vi "InstrumentSetup.vi"() -> ()   [LabVIEW 2013, in "InstrControl.lvclass"]
uses:
  InstrControl.lvclass
  ArduinoControl/ArduinoControl.lvclass
  Switching/Switching.lvclass
panel:
  in  "WayneKerr 6425 Configurations":T1={"RC Configuration"=0, "AC amplitude [V]"=0.1, "AC frequency [Hz]"=1000, "GPIB Address"="23"} {"RC Configuration" items=["serial", "parallel"]}
  in  "MUX & Matrix Configurations":T2={"GPIB address"="10", "Matrix address"="1", "Mux1 address"="4", "Mux2 address"="5", "Matrix used?"=FALSE, "Switching"=refnum, "Matrix X Channels"={"Bias Supply / SMU LO"=5, "Bias Supply / SMU HI"=6, "CV Box LO"=3, "CV Box HI"=4, "CV Box LO IN"=7, "CV Box HI IN"=8, "Volt meter LO"=1, "Volt meter HI"=2, "Mux1 C1"=9, "Mux1 C2"=10, "Mux2 C1"=11, "Mux2 C2"=12}}
  in  "WayneKerr 6440B Configurations":T1={"RC Configuration"=0, "AC amplitude [V]"=0.1, "AC frequency [Hz]"=1000, "GPIB Address"="23"} {"RC Configuration" items=["serial", "parallel"]}
  in  "Keithley 2000 Configurations":T3={"Range"=0, "Range Value"=100.0, "Function"=3, "GPIB Address"="19"} {"Function" items=["AC Current", "DC Current", "AC Voltage", "DC Voltage", "2W-Resistance", "4W-Resistance", "Period", "Frequency", "Temperature", "Diode", "Continuity"]; "Range Value" format="%#.2g"; "Range" items=["Auto", "Manual"]}
  in  "Arduino Configuration":T4={"VISA address"="COM24", "T sensor"=enum."SHT", "Arduino"=refnum}
  in  "Keithley 487 Configurations":T5={"Compliance"=0, "Range:"=0, "GPIB Address"="22"} {"Range:" items=["Autorange", "2nA", "20nA", "200nA", "2 microAmp", "20 microAmp", "200 microAmp", "2 milliAmp"]; "Compliance" items=["20µA", "2mA"]}
  in  "Keithley 2410 Configurations":T6={"Current Limit"=0.0001, "GPIB Address"="24"}
  in  "Keithley 6517 Configurations":T7={"Current Limit"=1, "GPIB Address"="27"} {"Current Limit" items=["OFF", "ON"]}
  in  "Keithley 236/237 Configurations":T8={"current \ncompliance level"=0.0001, "compliance/\nmeasurement range (auto:0)"=6, "GPIB Address"="16"} {"compliance/\nmeasurement range (auto:0)" items=["auto / auto", "1 nA / 1.1 V", "10 nA / 11 V", "100 nA / 110 V", "0.001 mA / 110 V", "0.01 mA / 110 V", "0.1 mA / 110 V", "1 mA / 110 V", "10 mA / 110 V", "100 mA / 110 V"]; "current \ncompliance level" format="%.4f"}
  in  "Default GPIB addresses":T9={"KE 487"="22", "KE 6517"="27", "WK 6425"="17", "KE 236 SMU"="16", "HP 4263B"="18", "KE 2000"="19", "KE 2410"="24", "WK 6440B"="23", "Matrix"="10"}
  # "DEFAULT VALUES FOR INSTRUMENT SETUP"
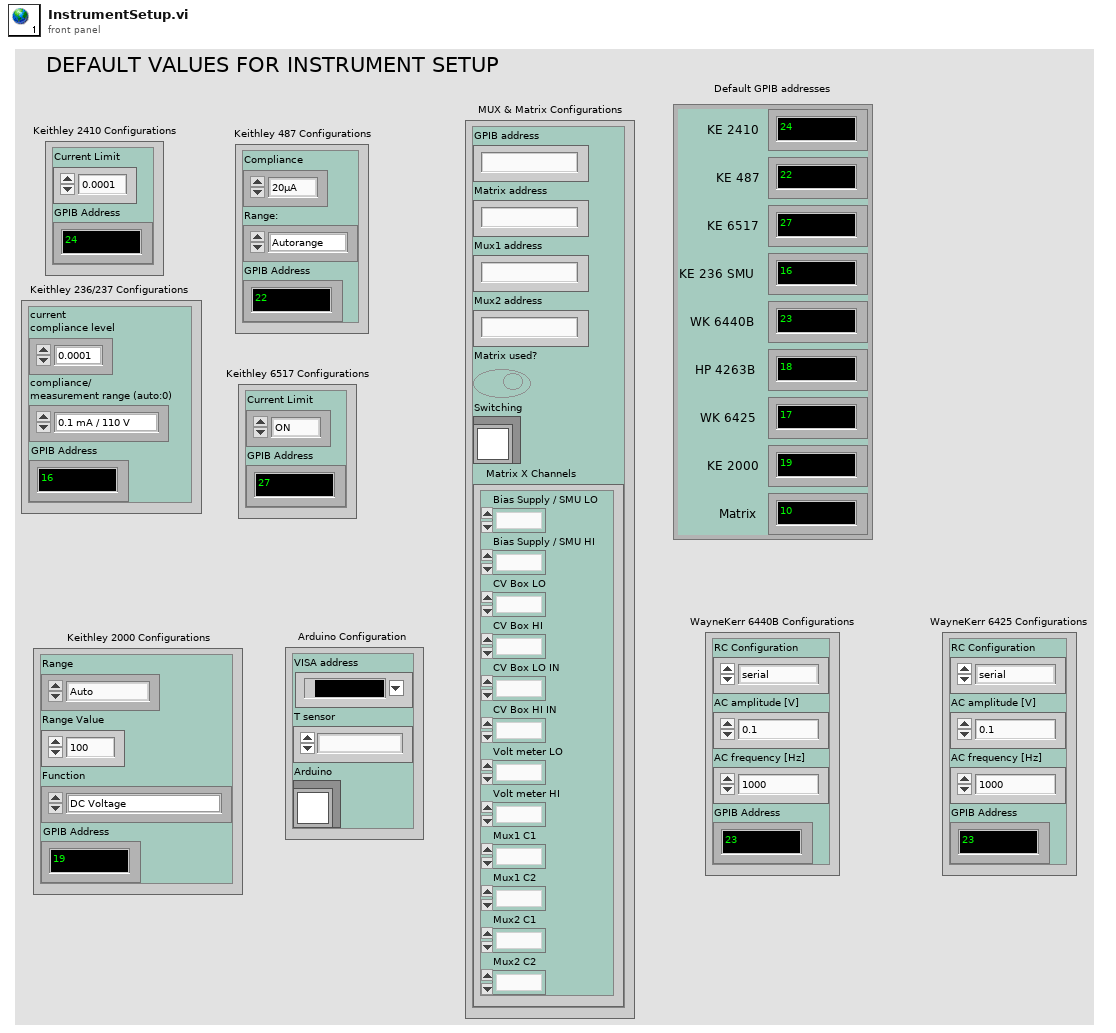
[diagram p1: front panel]
types:
  T1 = cluster{"RC Configuration":u16, "AC amplitude [V]":dbl, "AC frequency [Hz]":i32, "GPIB Address":string}
  T2 = cluster{"GPIB address":string, "Matrix address":string, "Mux1 address":string, "Mux2 address":string, "Matrix used?":bool, "Switching":refnum<class "Switching.lvclass">, "Matrix X Channels":cluster{"Bias Supply / SMU LO":i32, "Bias Supply / SMU HI":i32, "CV Box LO":i32, "CV Box HI":i32, "CV Box LO IN":i32, "CV Box HI IN":i32, "Volt meter LO":i32, "Volt meter HI":i32, "Mux1 C1":i32, "Mux1 C2":i32, "Mux2 C1":i32, "Mux2 C2":i32}}
  T3 = cluster{"Range":u16, "Range Value":dbl, "Function":u16, "GPIB Address":string}
  T4 = cluster{"VISA address":refnum<visa-resource-name>, "T sensor":enum16{"SHT", "DS"}, "Arduino":refnum<class "ArduinoControl.lvclass">}
  T5 = cluster{"Compliance":u16, "Range:":u16, "GPIB Address":string}
  T6 = cluster{"Current Limit":sgl, "GPIB Address":string}
  T7 = cluster{"Current Limit":u16, "GPIB Address":string}
  T8 = cluster{"current \ncompliance level":dbl, "compliance/\nmeasurement range (auto:0)":u16, "GPIB Address":string}
  T9 = cluster{"KE 487":string, "KE 6517":string, "WK 6425":string, "KE 236 SMU":string, "HP 4263B":string, "KE 2000":string, "KE 2410":string, "WK 6440B":string, "Matrix":string}
diagram:
